vi "thermistor converter.vi"() -> ()   [LabVIEW 2022 SP3]
panel:
  out "RT":dbl
  in  "R1":dbl
  in  "VT":dbl
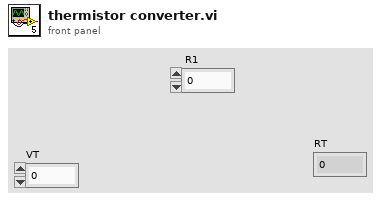
[diagram p1: front panel]
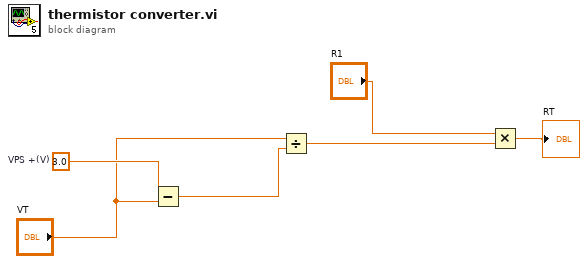
[diagram p0: block diagram]
diagram:
  w6 = 3.0  # VPS +(V)
  n1 = Subtract(x=w6, y="VT") -> (x-y=w4:dbl)
  n2 = Divide(x="VT", y=w4) -> (x/y=w1:dbl)
  n3 = Multiply(x="R1", y=w1) -> (x*y=→"RT":dbl)
